vi "set_center.vi"(8 "error in (no error)":errorcluster, 10 "center":refnum<class "SpaceVector.lvclass">, 11 "RoiGeneric in":refnum<class "RoiGeneric.lvclass">) -> (0 "error out":errorcluster, 3 "RoiGeneric out":refnum<class "RoiGeneric.lvclass">)   [LabVIEW 2010, in "RoiGeneric.lvclass"]
uses:
  RoiGeneric.lvclass
  common/classes/SpaceVector/SpaceVector/SpaceVector.lvclass
  RoiGeneric.lvclass/RoiGeneric.ctl
  common/classes/Box/Box/Box.lvclass
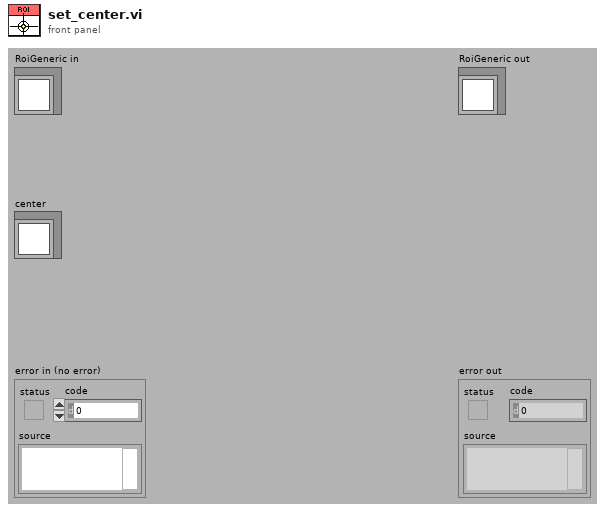
[diagram p1: front panel]
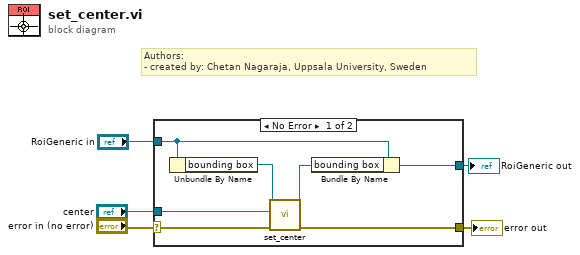
[diagram p0: block diagram]
diagram:
  # "Authors: \n- created by: Chetan Nagaraja, Uppsala University, Sweden"
  n1 = case shown="No Error" "error in (no error)" {
    selector: "error in (no error)" -> [w10 w14]
    tunnel: [w9 w14] -> w4
    tunnel: [w12 w13] -> w2
    tunnel: "RoiGeneric in" -> [w11 w13]
    tunnel: "center" -> [w6 _]
    frame No Error {
      n2 = Unbundle By Name(w11) -> ("bounding box"=w7:refnum<class "Box.lvclass">)
      n3 = call "set_center.vi"("error in (no error)"=w10, "new center"=w6, "Box in"=w7) -> ("error out"=w9:errorcluster, "Box out"=w8:refnum<class "Box.lvclass">)  [unwired: 7 in]
      n4 = Bundle By Name(cluster=w11, "bounding box"=w8) -> (w12:refnum<class "RoiGeneric.lvclass">)
    }
    frame Error {
    }
  }
  "error out" <- w4
  "RoiGeneric out" <- w2
